vi "Measure EQE_v2.vi"(6 "Skip cell?":bool, 8 "error in":errorcluster, 9 "Save data file path":string, 10 "Scan settings":T1={"J-V scan"=TRUE, "J-t scan"=FALSE, "Min voltage (V)"=0.0, "Max voltage (V)"=1.4, "Step (V)"=0.01, "Measurement delay (ms)"=10.0, "1st scan FB-SC"=TRUE, "Inverted structure"=FALSE, "Stabilisation time (s)"=0.0, "Stabilisation mode"=0, "Stabilisation value (V or A) "=0.0, "Step time (s)"=1.0, "Integration time"=0, "Repeat light scans"=FALSE, "Stabilisation in the dark?"=FALSE, "J-t Min (V)"=0.0, "J-t Max (V)"=1.4, "J-t Step (V)"=0.01, "Max. power stabilisation"=FALSE, "J-t 1st scan FB-SC"=TRUE, "J-t Inverted structure"=FALSE, "Max power tracking"=FALSE, "Vmp (V)"=0.7, "Total stabilisation time (s)"=100.0, "J-t best pixel only"=0, "Max power best pixel only"=0, "Vmp from J-V scan"=FALSE, "Intensity dependence"=FALSE, "P dep best pixel only"=0, "External quantum efficiency"=FALSE, "EQE best pixel only"=0, "WL min (nm)"=300.0, "WL max (nm)"=900.0, "WL step (nm)"=5.0, "Wait (ms)"=100.0, "No. of repeat scans"=2.0, "Only repeat for best pixel"=0, "Chopper Freq.  (Hz)"=90.0, "Time Constant (s)"=2.0, "Stabilisation time step (s)"=1.0, "Illumination conditions"=2, "Scan rate min (V/s)"=0.1, "Scan rate max (V/s)"=1.0, "No. of scan rate steps"=1.0, "Scan rate voltage step priority"=FALSE, "Scan rate measurement delay priority"=FALSE, "J-t Illumination conditions"=0, "White bias  (no. of suns)"=200.0, "Max P stab. Specific voltage"=FALSE} {"J-t Illumination conditions" items=["Light only", "Dark only", "Light then dark", "Dark then light"]; "No. of scan rate steps" min=1.0 step=1.0; "Illumination conditions" items=["Light only", "Dark only", "Light then dark", "Dark then light", "Light then dark then light", "Dark then light then dark"]; "Time Constant (s)" items=["0.003", "0.01", "0.03", "0.1", "0.3", "1", "3", "10", "30", "100"]; "Only repeat for best pixel" items=["only for best pixel", "for best 2 pixels", "for best 3 pixels", "for best 4 pixels", "for best 5 pixels", "for best 6 pixels", "for best 7 pixels", "for all pixels"]; "No. of repeat scans" min=1.0 step=1.0; "EQE best pixel only" items=["only the best pixel", "the best 2 pixel", "the best 3 pixel", "the best 4 pixel", "the best 5 pixel", "the best 6 pixel", "the best 7 pixel", "all pixels"]; "P dep best pixel only" items=["only the best pixel", "the best 2 pixels", "the best 3 pixels", "the best 4 pixels", "the best 5 pixels", "the best 6 pixels", "the best 7 pixels", "all pixels"]; "Max power best pixel only" items=["only the best pixel", "the best 2 pixels", "the best 3 pixels", "the best 4 pixels", "the best 5 pixels", "the best 6 pixels", "the best 7 pixels", "all pixels"]; "J-t best pixel only" items=["only the best pixel", "the best 2 pixels", "the best 3 pixels", "the best 4 pixels", "the best 5 pixels", "the best 6 pixels", "the best 7 pixels", "all pixels"]; "Integration time" items=["Fast", "Normal", "High Accuracy"]; "Stabilisation mode" items=["V", "I"]; "Measurement delay (ms)" min=10.0}) -> (0 "error out":errorcluster, 1 "Min WL (nm)":string, 2 "Max WL (nm)":string, 3 "EQE data file path":path)   [LabVIEW 2011]
uses:
  TypeDefs/Scan settings.ctl
  TypeDefs/Settings Boolean.ctl
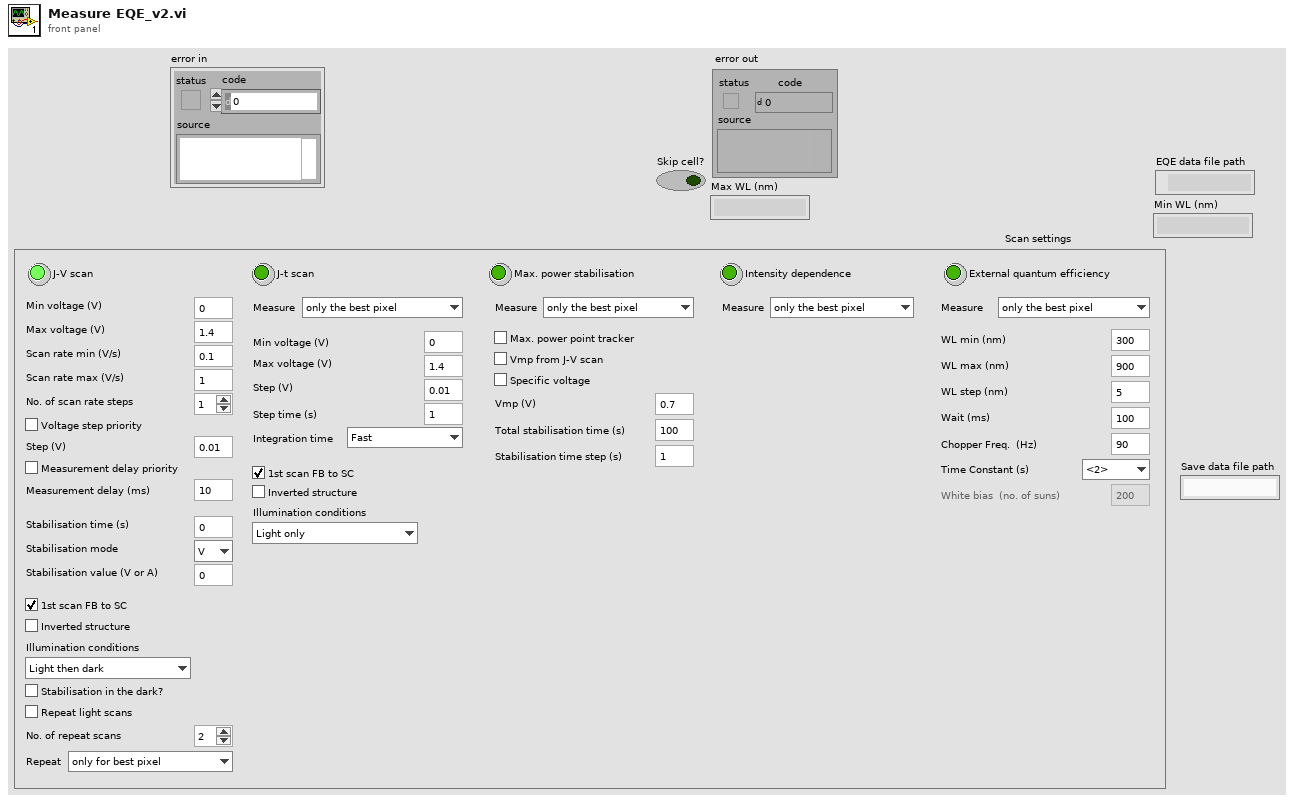
[diagram p1: front panel]
types:
  T1 = typedef "Scan settings.ctl" = cluster{"J-V scan":T2, "J-t scan":bool, "Min voltage (V)":dbl, "Max voltage (V)":dbl, "Step (V)":dbl, "Measurement delay (ms)":dbl, "1st scan FB-SC":bool, "Inverted structure":bool, "Stabilisation time (s)":dbl, "Stabilisation mode":u16, "Stabilisation value (V or A) ":dbl, "Step time (s)":dbl, "Integration time":u16, "Repeat light scans":bool, "Stabilisation in the dark?":bool, "J-t Min (V)":dbl, "J-t Max (V)":dbl, "J-t Step (V)":dbl, "Max. power stabilisation":bool, "J-t 1st scan FB-SC":bool, "J-t Inverted structure":bool, "Max power tracking":bool, "Vmp (V)":dbl, "Total stabilisation time (s)":dbl, "J-t best pixel only":u16, "Max power best pixel only":u16, "Vmp from J-V scan":bool, "Intensity dependence":bool, "P dep best pixel only":u16, "External quantum efficiency":bool, "EQE best pixel only":u16, "WL min (nm)":dbl, "WL max (nm)":dbl, "WL step (nm)":dbl, "Wait (ms)":dbl, "No. of repeat scans":dbl, "Only repeat for best pixel":u16, "Chopper Freq.  (Hz)":dbl, "Time Constant (s)":dbl, "Stabilisation time step (s)":dbl, "Illumination conditions":u16, "Scan rate min (V/s)":dbl, "Scan rate max (V/s)":dbl, "No. of scan rate steps":dbl, "Scan rate voltage step priority":bool, "Scan rate measurement delay priority":bool, "J-t Illumination conditions":u16, "White bias  (no. of suns)":dbl, "Max P stab. Specific voltage":bool}
  T2 = typedef "Settings Boolean.ctl" = bool
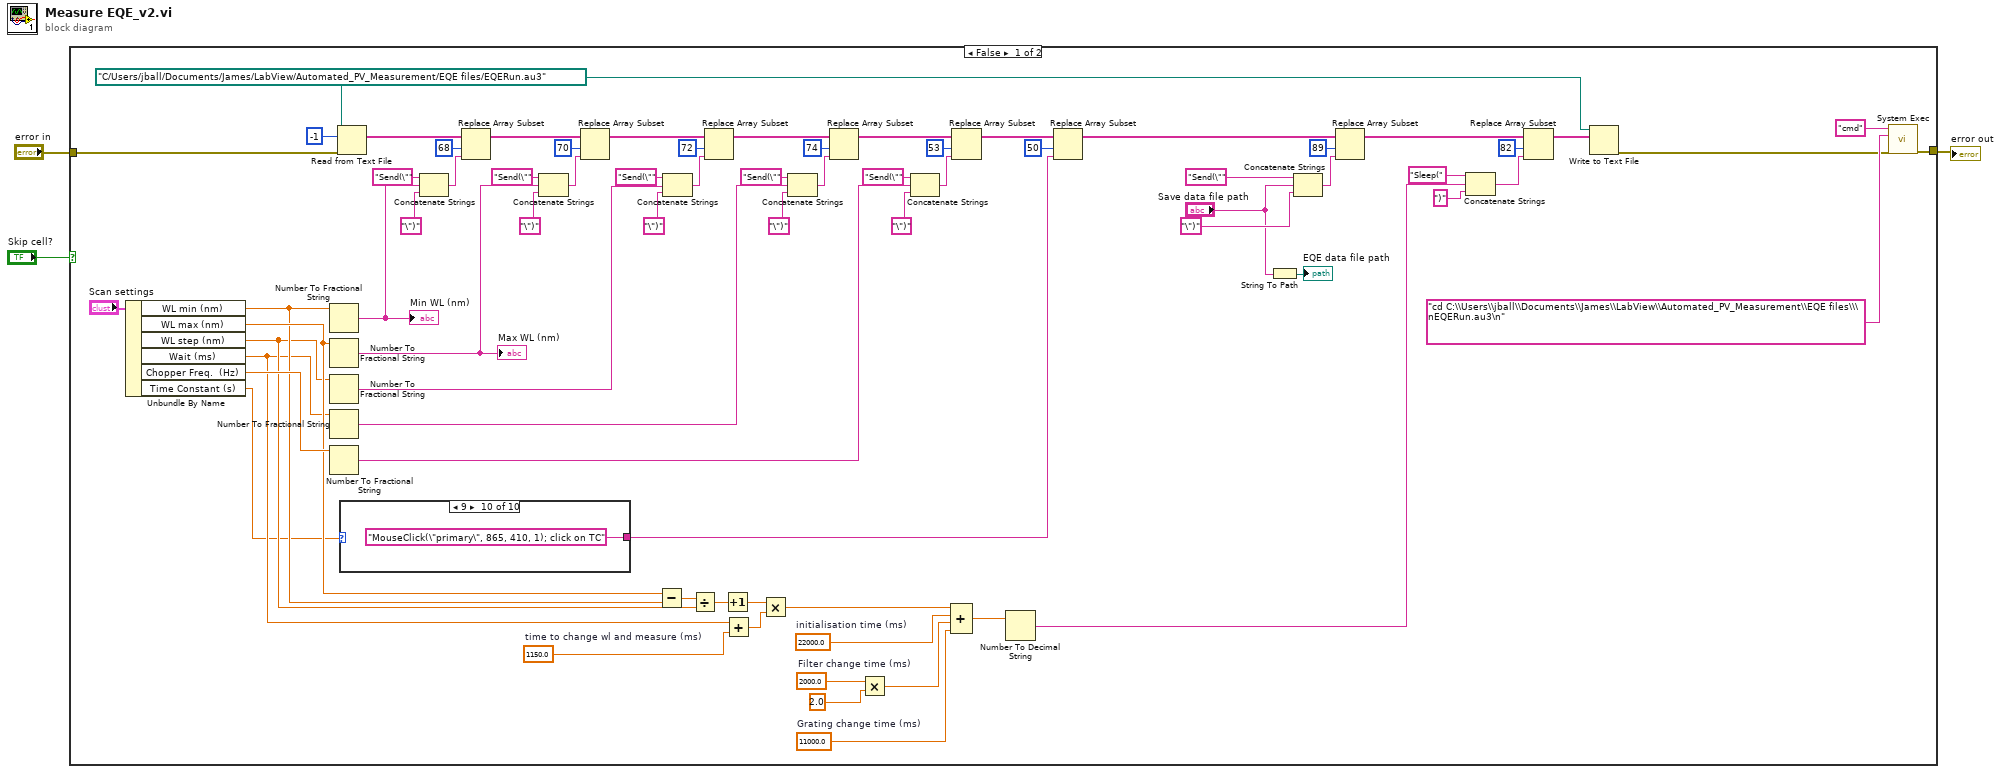
[diagram p0: block diagram]
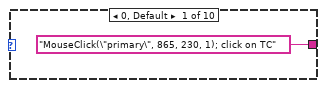
[diagram p2: hidden frame]
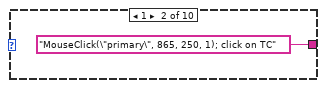
[diagram p3: hidden frame]
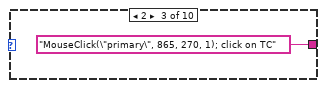
[diagram p4: hidden frame]
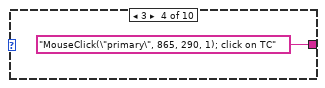
[diagram p5: hidden frame]
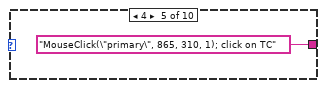
[diagram p6: hidden frame]
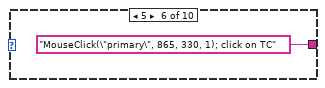
[diagram p7: hidden frame]
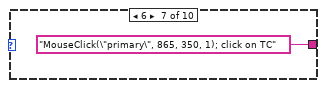
[diagram p8: hidden frame]
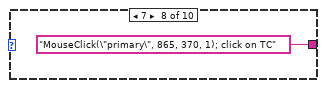
[diagram p9: hidden frame]
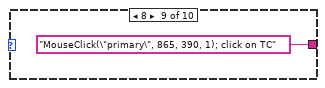
[diagram p10: hidden frame]
diagram:
  n1 = case shown="False" "Skip cell?" {
    tunnel: [w40 w87] -> w2
    tunnel: "error in" -> [w39 w87]
    frame False {
      w49 = 11000.0  # Grating change time (ms)
      w52 = 2000.0  # Filter change time (ms)
      w53 = 22000.0  # initialisation time (ms)
      w57 = 1150.0  # time to change wl and measure (ms)
      w42 = path "C:/Users/jball/Documents/James/LabView/Automated_PV_Measurement/EQE files/EQERun.au3" ("file (use dialog)")
      n2 = Unbundle By Name("Scan settings") -> ("WL min (nm)"=w62:dbl, "WL max (nm)"=w63:dbl, "WL step (nm)"=w60:dbl, "Wait (ms)"=w56:dbl, "Chopper Freq.  (Hz)"=w67:dbl, "Time Constant (s)"=w8:dbl)
      n3 = Number To Fractional String(number=w62) -> (F-format string=w33:string)  [unwired: 3 in]
      "Min WL (nm)" <- w33
      n4 = Number To Fractional String(number=w63) -> (F-format string=w27:string)  [unwired: 3 in]
      "Max WL (nm)" <- w27
      n5 = Number To Fractional String(number=w60) -> (F-format string=w21:string)  [unwired: 3 in]
      n6 = Number To Fractional String(number=w56) -> (F-format string=w15:string)  [unwired: 3 in]
      n7 = Number To Fractional String(number=w67) -> (F-format string=w9:string)  [unwired: 3 in]
      n8 = Read from Text File(file (use dialog)=w42, count=-1, error in=w39) -> (text=w34:string[])  [unwired: 1 in, 3 out]
      n9 = case shown="9" w8 {
        tunnel: ["MouseClick(\"primary\", 865, 230, 1); click on TC" ("string") "MouseClick(\"primary\", 865, 250, 1); click on TC" ("string") "MouseClick(\"primary\", 865, 270, 1); click on TC" ("string") "MouseClick(\"primary\", 865, 290, 1); click on TC" ("string") "MouseClick(\"primary\", 865, 310, 1); click on TC" ("string") "MouseClick(\"primary\", 865, 330, 1); click on TC" ("string") "MouseClick(\"primary\", 865, 350, 1); click on TC" ("string") "MouseClick(\"primary\", 865, 370, 1); click on TC" ("string") "MouseClick(\"primary\", 865, 390, 1); click on TC" ("string") "MouseClick(\"primary\", 865, 410, 1); click on TC" ("string")] -> w7
        frame 0, Default {
        }
        frame 1 {
        }
        frame 2 {
        }
        frame 3 {
        }
        frame 4 {
        }
        frame 5 {
        }
        frame 6 {
        }
        frame 7 {
        }
        frame 8 {
        }
        frame 9 {
        }
      }
      n10 = Concatenate Strings("Send(\"" ("string"), w33, "\")" ("string")) -> (w35:string)
      n11 = Replace Array Subset(array=w34, new element=w35, index=68) -> (w28:string[])
      n12 = Concatenate Strings("Send(\"" ("string"), w27, "\")" ("string")) -> (w29:string)
      n13 = Replace Array Subset(array=w28, new element=w29, index=70) -> (w22:string[])
      n14 = Subtract(x=w63, y=w62) -> (x-y=w61:dbl)
      n15 = Concatenate Strings("Send(\"" ("string"), w21, "\")" ("string")) -> (w23:string)
      n16 = Divide(x=w61, y=w60) -> (x/y=w59:dbl)
      n17 = Replace Array Subset(array=w22, new element=w23, index=72) -> (w16:string[])
      n18 = Increment(x=w59) -> (x+1=w58:dbl)
      n19 = Add(x=w56, y=w57) -> (x+y=w55:dbl)
      n20 = Multiply(x=w58, y=w55) -> (x*y=w54:dbl)
      n21 = Concatenate Strings("Send(\"" ("string"), w15, "\")" ("string")) -> (w17:string)
      n22 = Replace Array Subset(array=w16, new element=w17, index=74) -> (w10:string[])
      n23 = Multiply(x=w52, y=2.0) -> (x*y=w50:dbl)
      n24 = Concatenate Strings("Send(\"" ("string"), w9, "\")" ("string")) -> (w11:string)
      n25 = Compound Arithmetic op=ADD(w54, w53, w50, w49) -> (w48:dbl)
      n26 = Replace Array Subset(array=w10, new element=w11, index=53) -> (w6:string[])
      n27 = Number To Decimal String(number=w48) -> (decimal integer string=w46:string)  [unwired: 1 in]
      n28 = Replace Array Subset(array=w6, new element=w7, index=50) -> (w4:string[])
      n29 = String To Path(string="Save data file path") -> (path=→"EQE data file path":path)
      n30 = Concatenate Strings("Send(\"" ("string"), "Save data file path", "\")" ("string")) -> (w71:string)
      n31 = Replace Array Subset(array=w4, new element=w71, index=89) -> (w64:string[])
      n32 = Concatenate Strings("Sleep(" ("string"), w46, ")" ("string")) -> (w44:string)
      n33 = Replace Array Subset(array=w64, new element=w44, index=82) -> (w43:string[])
      n34 = Write to Text File(file (use dialog)=w42, text=w43) -> (error out=w41:errorcluster)  [unwired: 2 in, 2 out]
      n35 = call <vilib>:"System Exec.vi"("error in (no error)"=w41, "standard input"="cd C:\\Users\\jball\\Documents\\James\\LabView\\Automated_PV_Measurement\\EQE files\\\nEQERun.au3\n", "command line"="cmd") -> ("error out"=w40:errorcluster)  [unwired: 5 in, 3 out]
    }
    frame True {
    }
  }
  "error out" <- w2
